vi "Write Message.vi"(8 "error in (no error)":errorcluster, 10 "Message":string, 11 "Send Log Message MSG in":refnum<class "Send Log Message MSG.lvclass">) -> (0 "error out":errorcluster, 3 "Send Log Message MSG out":refnum<class "Send Log Message MSG.lvclass">)   [LabVIEW 2014, in "Controller.lvlib" / "Send Log Message MSG.lvclass"]
uses:
  Send Log Message MSG.lvclass
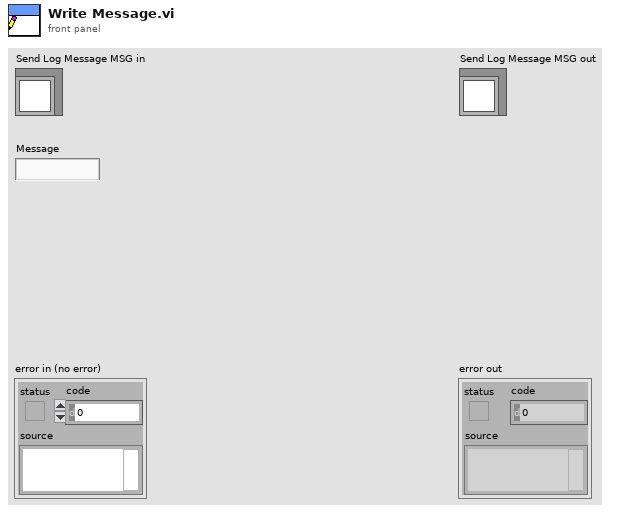
[diagram p1: front panel]
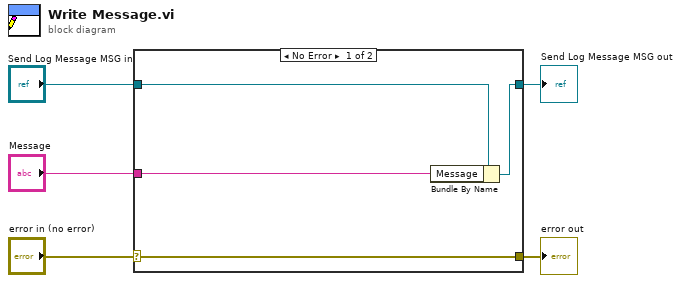
[diagram p0: block diagram]
diagram:
  n1 = case shown="No Error" "error in (no error)" {
    selector: "error in (no error)" -> [w9 w10]
    tunnel: [w9 w10] -> w4
    tunnel: [w7 w11] -> w2
    tunnel: "Send Log Message MSG in" -> [w8 w11]
    tunnel: "Message" -> [w6 _]
    frame No Error {
      n2 = Bundle By Name(cluster=w8, "Message"=w6) -> (w7:refnum<class "Send Log Message MSG.lvclass">)
    }
    frame Error {
    }
  }
  "error out" <- w4
  "Send Log Message MSG out" <- w2
